vi "niVNA_Auto Port Extend.vi"(7 "Pins":string[](array[string])=["RF1", "RF2"], 8 "error in (no error)":errorcluster, 11 "Semiconductor Module Context":T1) -> (0 "error out":errorcluster, 3 "Semiconductor Module Context Out":T1)   [LabVIEW 2013]
uses:
  <vilib>/NI_TestStand_SemiconductorModule/NI_TestStand_Semiconductor_Module.lvlibp/PinMap/General/SemiconductorModuleContext.ctl
  Pin Map API/VNA Custom Instrument.lvlib
  <vilib>/NI_TestStand_SemiconductorModule/NI_TestStand_Semiconductor_Module.lvlibp
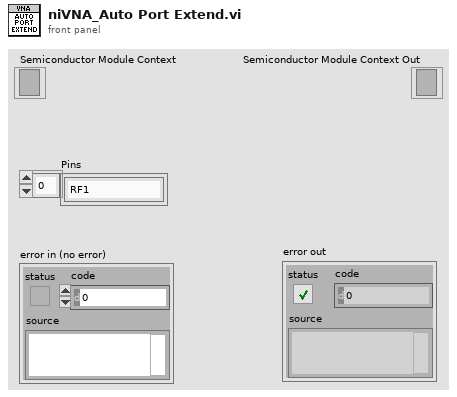
[diagram p1: front panel]
types:
  T1 = typedef "NI_TestStand_Semiconductor_Module.lvlibp/SemiconductorModuleContext.ctl" = refnum<k7>
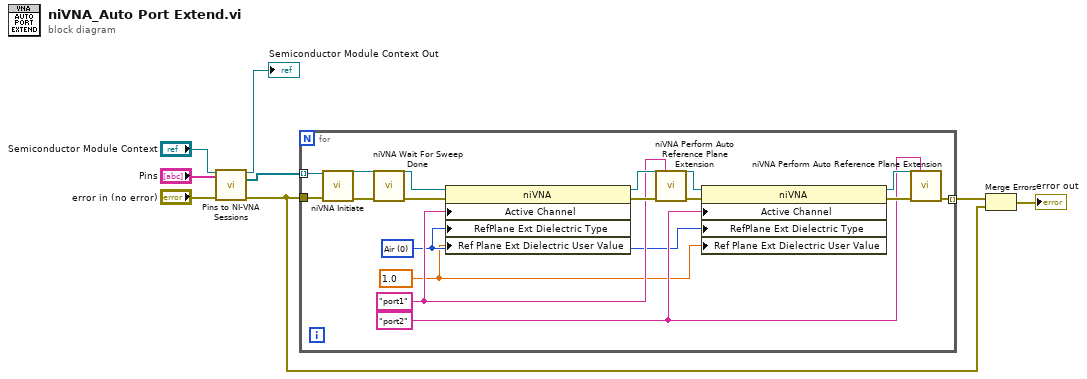
[diagram p0: block diagram]
diagram:
  n1 = call "Pins to NI-VNA Sessions.vi"("Semiconductor Module Context"="Semiconductor Module Context", "Pins"="Pins", "error in (no error)"="error in (no error)") -> ("Semiconductor Module Context Out"=→"Semiconductor Module Context Out":T1, "Instrument Sessions"=w5:refnum<k15>[], "error out"=w2:errorcluster)  [unwired: 8 in, 2 out]
  n2 = for {
    tunnel: w2 -> [w11]
    tunnel: w5 -> [w10] mode=indexing
    tunnel: [w9] -> w3 mode=indexing
    w12 = 1.0 ("RPE Dielectric User Value")
    w13 = 0 items=["Air", "Polyethylene", "Teflon", "Micro Teflon", "User Value"] ("RPE Dielectric Type")
    w14 = "port2" ("port")
    w15 = "port1" ("port")
    n3 = call <instrlib>:"niVNA Initiate.vi"("instrument handle"=w10, "error in"=w11) -> ("instrument handle out"=w25:refnum<k15>, "error out"=w22:errorcluster)  [unwired: 12 in]
    n4 = call <instrlib>:"niVNA Wait For Sweep Done.vi"("instrument handle"=w25, "error in"=w22) -> ("instrument handle out"=w24:refnum<k15>, "error out"=w23:errorcluster)  [unwired: 12 in]
    n5 = property class="niVNA"(reference=w24, error in=w23, "Active Channel"=w15, "RefPlane Ext Dielectric Type"=w13, "Ref Plane Ext Dielectric User Value"=w12) -> (reference out=w20:refnum<k15>, error out=w21:errorcluster)
    n6 = call <instrlib>:"niVNA Perform Auto Reference Plane Extension.vi"("instrument handle"=w20, "port"=w15, "error in"=w21) -> ("instrument handle out"=w18:refnum<k15>, "error out"=w19:errorcluster)  [unwired: 11 in]
    n7 = property class="niVNA"(reference=w18, error in=w19, "Active Channel"=w14, "RefPlane Ext Dielectric Type"=w13, "Ref Plane Ext Dielectric User Value"=w12) -> (reference out=w16:refnum<k15>, error out=w17:errorcluster)
    n8 = call <instrlib>:"niVNA Perform Auto Reference Plane Extension.vi"("instrument handle"=w16, "port"=w14, "error in"=w17) -> ("error out"=w9:errorcluster)  [unwired: 11 in, 1 out]
  }
  n9 = Merge Errors(w3, w2) -> (→"error out":errorcluster)
